vi "fallout_terminal_hacker.vi"() -> ()   [LabVIEW 2018]
uses:
  <userlib>/_OpenG.lib/string/string.llb/Trim Whitespace (String)__ogtk.vi
panel:
  out "It Could Be":string[](array[string])
  in  "Submit":bool
  in  "Likeness":i32
  in  "Word Tried":string
  in  "Words Available":string="shot\nhurt\nsell\ngive\nsure\ngear\nsent\nfire\nglow\nweek\nones\nsick"
  # "Instructions:\n1: Type into \"Words Available\" the words available from\nthe terminal from Fallout.  Use a new line for each word.\n\n2: Hit the Run arrow to start this program."
  # "3: In the terminal in Fallout, select one of the\nwords available from \"It Could Be\" here.  It will\ntell you the \"Likeness\" between what you\nselected and what the actual password is.  Enter\nthat word in \"Word Tried\" below and the likeness\nin \"Likeness\" below and press Submit."
  # "\"It Could Be\" indicator below\nreduces to possible words.\nFrom this list of possible words,\nrepeat step 3."
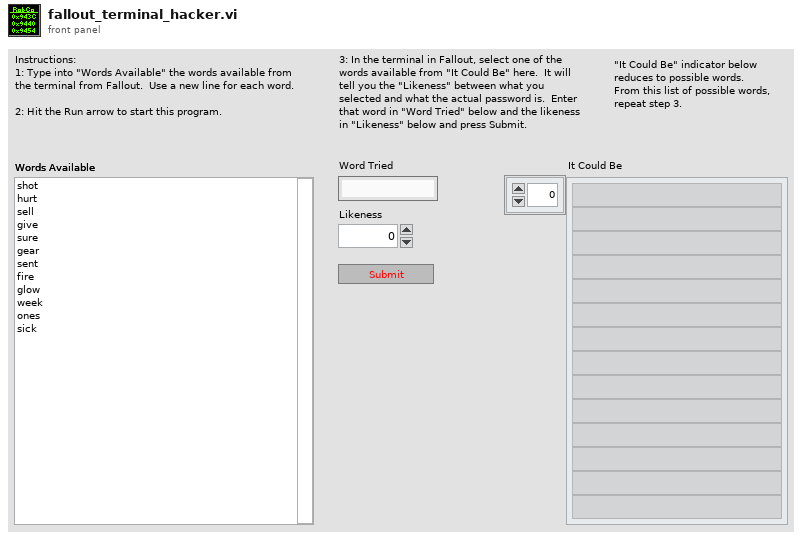
[diagram p1: front panel]
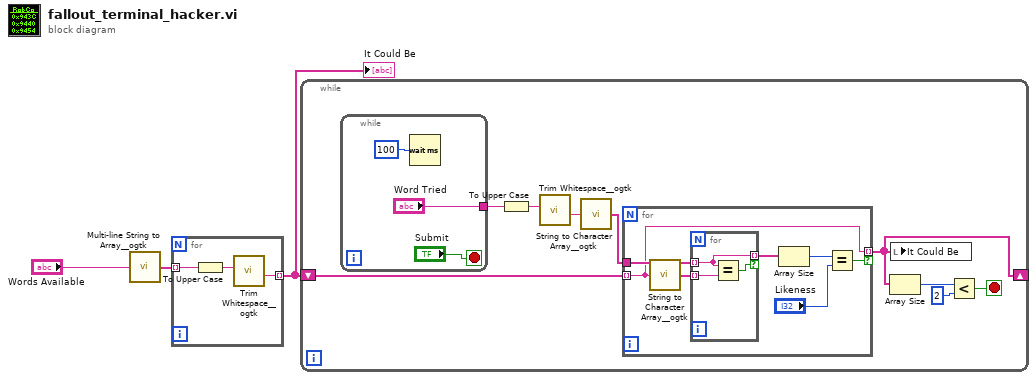
[diagram p0: block diagram]
diagram:
  n1 = call <userlib>:"Multi-line String to Array__ogtk.vi"("string"="Words Available") -> ("lines"=w2:string[])
  n2 = for {
    tunnel: w2 -> [w6] mode=indexing
    tunnel: [w4] -> w1 mode=indexing
    n3 = To Upper Case(1:w6) -> (0:w5:string)
    n4 = call-poly <userlib>:"Trim Whitespace__ogtk.vi"("String in"=w5) -> ("String out"=w4:string)  [unwired: 6 in]
  }
  "It Could Be" <- w1
  n5 = while {
    shift-right: [w10] -> _
    shift-left: w1 -> [w11]
    stop <- w7 stop-if-true
    n6 = while {
      tunnel: ["Word Tried"] -> w12
      stop <- "Submit" stop-if-true
      n7 = Wait (ms)(milliseconds to wait=u32 100) -> ()  [unwired: 1 out]
    }
    n8 = To Upper Case(1:w12) -> (0:w14:string)
    n9 = call-poly <userlib>:"Trim Whitespace__ogtk.vi"("String in"=w14) -> ("String out"=w13:string)  [unwired: 6 in]
    n10 = call <userlib>:"String to Character Array__ogtk.vi"("Input String"=w13) -> ("Character Array"=w15:string[])
    n11 = for {
      tunnel: w15 -> [w25]
      tunnel: w11 -> [w19] mode=indexing
      tunnel: [w19] -> w10 mode=indexing if=w21
      n12 = call <userlib>:"String to Character Array__ogtk.vi"("Input String"=w19) -> ("Character Array"=w20:string[])
      n13 = for {
        tunnel: w20 -> [w27] mode=indexing
        tunnel: w25 -> [w28] mode=indexing
        tunnel: [w28] -> w22 mode=indexing if=w26
        n14 = Equal?(x=w28, y=w27) -> (x = y?=w26:bool)
      }
      n15 = Array Size(array=w22) -> (size(s)=w23:i32)
      n16 = Equal?(x=w23, y="Likeness") -> (x = y?=w21:bool)
    }
    n17 = Array Size(array=w10) -> (size(s)=w9:i32)
    n18 = local write "It Could Be"(w10) -> ()
    n19 = Less?(x=w9, y=2) -> (x < y?=w7:bool)
  }
